vi "readFromXML.vi"(8 "error in (no error)":errorcluster, 10 "XMLin":string="<RADecParameters>\n  <declination>\n    <degreesDec>46</degreesDec>\n    <minutesArc>31</minutesArc> \n    <secondsArc>16</secondsArc>\n  </declination>\n  <equinoxPrefix>J</equinoxPrefix>\n  <equinoxYear>2000</equinoxYear>\n  <frame>FK5</frame>\n  <ra>\n    <hours>16</hours>  \n    <minutesTime>11</minutesTime>\n    <secondsTime>9</secondsTime>\n  </ra>\n</RADecParameters>", 11 "RADecParameters in":refnum<class "RADecParameters.lvclass">) -> (0 "error out":errorcluster, 3 "RADecParameters out":refnum<class "RADecParameters.lvclass">)   [LabVIEW 2014, in "TCSDataDefinitions.lvlib" / "TCSCommand.lvlib" / "TargetConfiguration.lvlib" / "Target.lvlib" / "FixedTarget.lvlib" / "RADecParameters.lvclass"]
uses:
  RADecParameters.lvclass
  Declination/Declination.lvclass
  TCSPublicStatus/CurrentTimes/ClockTimes/ClockTimes.lvclass
  Enumerations/EquinoxPrefix.ctl
  Enumerations/FrameValues.ctl
  RADecParameters.lvclass/RADecParameters.ctl
  <userlib>/Common/XML/XMLParser/XMLParser.lvclass
  FixedTarget.lvlib
panel:
  out "frame":T1
  out "equinoxYear":dbl
  out "equinoxPrefix":T2
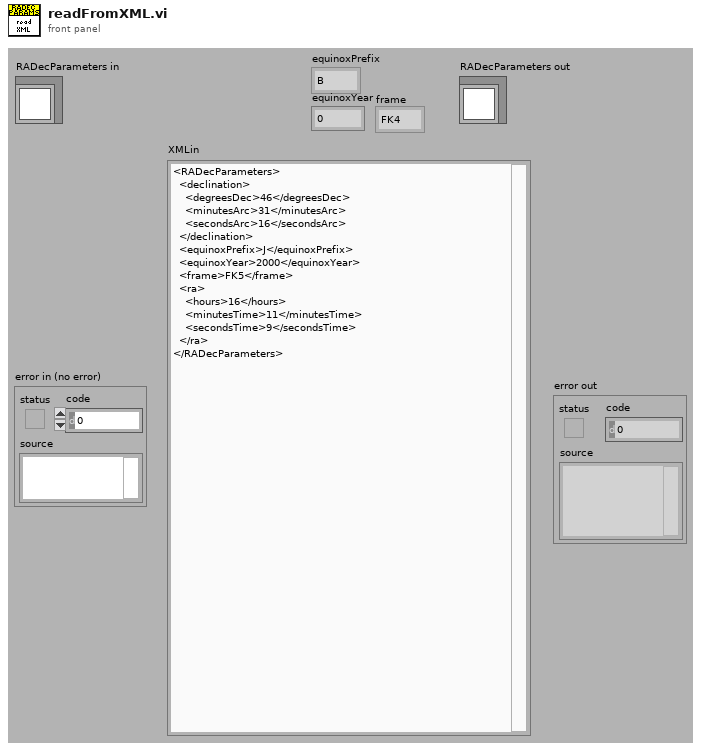
[diagram p1: front panel]
types:
  T1 = typedef "TCSDataDefinitions.lvlib/TCSCommand.lvlib/TargetConfiguration.lvlib/Target.lvlib/FixedTarget.lvlib/FrameValues.ctl" = enum16{"FK4", "FK5", "APPT", "GAPPT", "AZEL"}
  T2 = typedef "TCSDataDefinitions.lvlib/TCSCommand.lvlib/TargetConfiguration.lvlib/Target.lvlib/FixedTarget.lvlib/EquinoxPrefix.ctl" = enum16{"B", "J"}
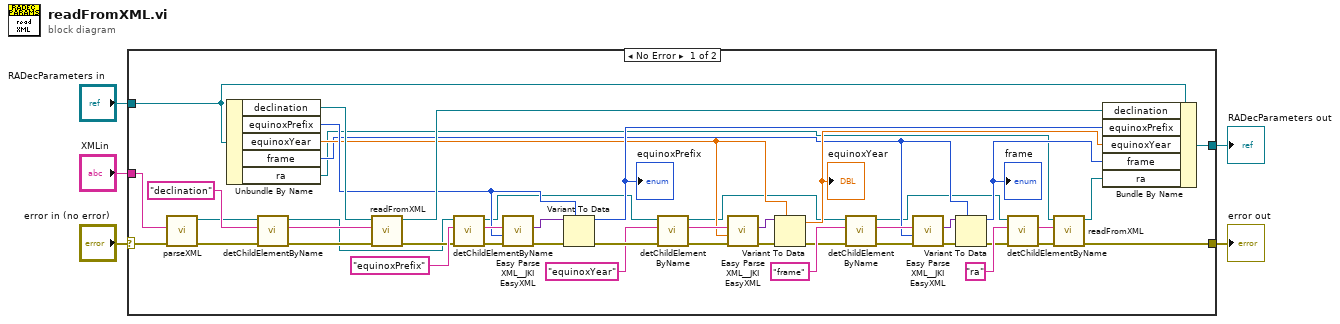
[diagram p0: block diagram]
diagram:
  n1 = case shown="No Error" "error in (no error)" {
    selector: "error in (no error)" -> [w49 w53]
    tunnel: [w11 w53] -> w4
    tunnel: [w46 w52] -> w2
    tunnel: "RADecParameters in" -> [w47 w52]
    tunnel: "XMLin" -> [w51 _]
    frame No Error {
      n2 = call <userlib>:"parseXML.vi"("error in (no error)"=w49, "XMLString in"=w51) -> ("error out"=w50:errorcluster, "Element out"=w10:refnum<class "XMLParser.lvclass">)  [unwired: 8 in]
      n3 = Unbundle By Name(w47) -> ("declination"=w45:refnum<class "Declination.lvclass">, "equinoxPrefix"=w35:T2, "equinoxYear"=w25:dbl, "frame"=w17:T1, "ra"=w13:refnum<class "ClockTimes.lvclass">)
      n4 = call <userlib>:"detChildElementByName.vi"("error in (no error)"=w50, "childName"="declination" ("ChildName"), "Element in"=w10) -> ("error out"=w42:errorcluster, "childXML"=w44:string, "Element out"=w9:refnum<class "XMLParser.lvclass">)  [unwired: 5 in, 1 out]
      n5 = call-dynamic "readFromXML.vi"("error in (no error)"=w42, "XML in"=w44, "Declination in"=w45) -> ("error out"=w38:errorcluster, "Declination out"=w43:refnum<class "Declination.lvclass">)  [unwired: 7 in]
      n6 = call <userlib>:"detChildElementByName.vi"("error in (no error)"=w38, "childName"="equinoxPrefix" ("ChildName"), "Element in"=w9) -> ("error out"=w37:errorcluster, "childXML"=w39:string, "Element out"=w8:refnum<class "XMLParser.lvclass">)  [unwired: 5 in, 1 out]
      n7 = call <vilib>:"Easy Parse XML__JKI EasyXML.vi"("error in (no error)"=w37, "LabVIEW Data (Type)"=w35, "XML String"=w39) -> ("error out"=w41:errorcluster, "LabVIEW Data"=w29:variant)  [unwired: 7 in]
      n8 = Variant To Data(error in=w41, type=w35, Variant=w29) -> (data=w34:T2, error out=w36:errorcluster)
      "equinoxPrefix" <- w34
      n9 = call <userlib>:"detChildElementByName.vi"("error in (no error)"=w36, "childName"="equinoxYear" ("ChildName"), "Element in"=w8) -> ("error out"=w27:errorcluster, "childXML"=w28:string, "Element out"=w7:refnum<class "XMLParser.lvclass">)  [unwired: 5 in, 1 out]
      n10 = call <vilib>:"Easy Parse XML__JKI EasyXML.vi"("error in (no error)"=w27, "LabVIEW Data (Type)"=w25, "XML String"=w28) -> ("error out"=w31:errorcluster, "LabVIEW Data"=w30:variant)  [unwired: 7 in]
      n11 = Variant To Data(error in=w31, type=w25, Variant=w30) -> (data=w24:dbl, error out=w26:errorcluster)
      "equinoxYear" <- w24
      n12 = call <userlib>:"detChildElementByName.vi"("error in (no error)"=w26, "childName"="frame" ("ChildName"), "Element in"=w7) -> ("error out"=w19:errorcluster, "childXML"=w20:string, "Element out"=w6:refnum<class "XMLParser.lvclass">)  [unwired: 5 in, 1 out]
      n13 = call <vilib>:"Easy Parse XML__JKI EasyXML.vi"("error in (no error)"=w19, "LabVIEW Data (Type)"=w17, "XML String"=w20) -> ("error out"=w22:errorcluster, "LabVIEW Data"=w21:variant)  [unwired: 7 in]
      n14 = Variant To Data(error in=w22, type=w17, Variant=w21) -> (data=w16:T1, error out=w18:errorcluster)
      "frame" <- w16
      n15 = call <userlib>:"detChildElementByName.vi"("error in (no error)"=w18, "childName"="ra" ("ChildName"), "Element in"=w6) -> ("error out"=w14:errorcluster, "childXML"=w15:string)  [unwired: 5 in, 2 out]
      n16 = call-dynamic "readFromXML.vi"("error in (no error)"=w14, "XML in"=w15, "ClockTimes in"=w13) -> ("error out"=w11:errorcluster, "ClockTimes out"=w12:refnum<class "ClockTimes.lvclass">)  [unwired: 7 in]
      n17 = Bundle By Name(cluster=w47, "declination"=w43, "equinoxPrefix"=w34, "equinoxYear"=w24, "frame"=w16, "ra"=w12) -> (w46:refnum<class "RADecParameters.lvclass">)
    }
    frame Error {
    }
  }
  "error out" <- w4
  "RADecParameters out" <- w2
